vi "Get Timestamp.vi"(8 "error in":errorcluster, 11 "CANopen Message in":refnum<class "CANopen Message.lvclass">) -> (0 "error out":errorcluster, 2 "Timestamp":timestamp format="%<%x %.3X>T", 3 "CANopen Message out":refnum<class "CANopen Message.lvclass">)   [LabVIEW 2020, in "CANopen.lvlib" / "CANopen Message.lvclass"]
uses:
  CANopen Message.lvclass
  CANopen Message.lvclass/CANopen Message.ctl
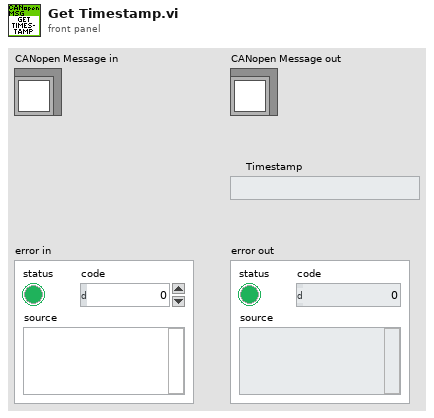
[diagram p1: front panel]
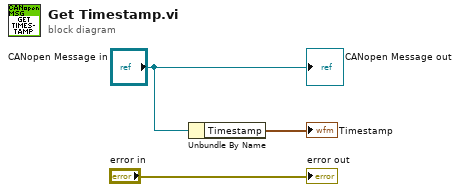
[diagram p0: block diagram]
diagram:
  n1 = Unbundle By Name("CANopen Message in") -> ("Timestamp"=→"Timestamp":timestamp)
  "CANopen Message out" <- "CANopen Message in"
  "error out" <- "error in"
